vi "Configure Measurement Time.vi"(0 "VISA resource name":refnum<visa-resource-name>, 5 "Measurement Time (6 PLC)":dbl=6.0, 11 "error in (no error)":errorcluster) -> (4 "VISA resource name out":refnum<visa-resource-name>, 15 "error out":errorcluster)   [LabVIEW 2024, in "Keithley 648X Series.lvlib"]
doc: "Sets the integration time of the A/D converter. This is the period of time the input signal is measured. The integration time affects the amount of reading noise as well as the ultimate reading rate of the instrument."
uses:
  <instrlib>/Keithley 648X Series/Keithley 648X Series.lvlib
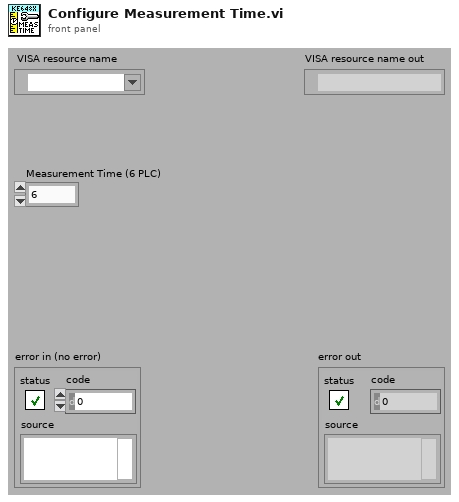
[diagram p1: front panel]
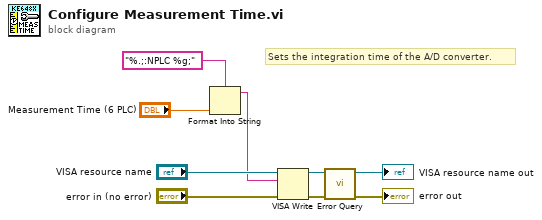
[diagram p0: block diagram]
diagram:
  # "Sets the integration time of the A/D converter."
  n1 = Format Into String(format string="%.;:NPLC %g;", "Measurement Time (6 PLC)") -> (resulting string=w1:string)  [unwired: 2 in, 1 out]
  n2 = VISA Write(VISA resource name="VISA resource name", write buffer=w1, error in (no error)="error in (no error)") -> (VISA resource name out=w5:refnum<visa-resource-name>, error out=w4:errorcluster)  [unwired: 1 out]
  n3 = call <instrlib>:"Error Query.vi"("error in (no error)"=w4, "VISA resource name"=w5) -> ("error out"=→"error out":errorcluster, "VISA resource name out"=→"VISA resource name out":refnum<visa-resource-name>)  [unwired: 6 in, 2 out]
